vi "Handle Last Ack Core.vi"(4 "error in (no error)":errorcluster, 6 "Last Ack":refnum<class "Last Ack.lvclass">, 7 "Server in":refnum<class "Server.lvclass">) -> (0 "error out":errorcluster, 3 "Server out":refnum<class "Server.lvclass">)   [LabVIEW 2020, in "Server.lvlib" / "Server.lvclass"]
doc: "(<B>Filename</B>: Actor Framework.lvlib:Actor.lvclass:Handle Last Ack Core.vi)\n\nDefines how the caller actor responds to the Last Ack message from a nested actor. The Last Ack message is the final message a nested actor sends to its caller before it shuts down. The message contains information about the final state of the nested actor.\n\nBy default, this method does nothing except return any error the nested actor sent. A descendant class may override this method to define behavior."
uses:
  Server.lvclass
  <vilib>/ActorFramework/LastAck/Last Ack.lvclass
  C:/Program Files/National Instruments/LabVIEW 2020/vi.lib/ActorFramework/Actor/Actor.lvclass
  <vilib>/ActorFramework/Actor/Actor.lvclass/Actor.ctl
  <vilib>/ActorFramework/Message Enqueuer/Message Enqueuer.lvclass/Message Enqueuer.ctl
  Server.lvclass/Server.ctl
  Chat Window Model/Chat Window Model Messages/Update Online List Msg/Update Online List Msg.lvclass/Update Online List Msg.ctl
  Chat Window Model/Chat Window Model Messages/Update Status Log Msg/Update Status Log Msg.lvclass/Update Status Log Msg.ctl
  Server Messages/Enable Controls Msg/Enable Controls Msg.lvclass/Enable Controls Msg.ctl
  <vilib>/ActorFramework/Message Enqueuer/Init from Existing Queue.vi
  <vilib>/ActorFramework/Message Enqueuer/Enqueue.vi
  Chat Window Model/Chat Window Model Messages/Update Online List Msg/Update Online List Msg.lvclass
  C:/Program Files/National Instruments/LabVIEW 2020/vi.lib/ActorFramework/Message/Message.lvclass
  Chat Window Model/Chat Window Model Messages/Update Status Log Msg/Update Status Log Msg.lvclass
  Server Messages/Enable Controls Msg/Enable Controls Msg.lvclass
  <vilib>/ActorFramework/Message Priority Queue/Priority Enqueue.vi
  <vilib>/ActorFramework/Message Enqueuer/Message Enqueuer.lvclass
  <vilib>/ActorFramework/Actor/Actor.lvclass
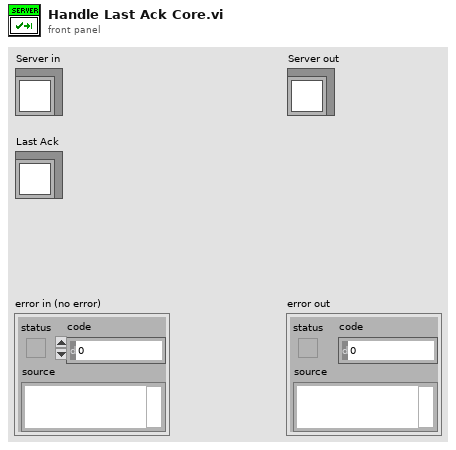
[diagram p1: front panel]
types:
  T1 = enum8{"Enabled", "Disabled", "Disabled and Grayed Out"}
  T2 = map{string, cluster{"Enqueuer":refnum<class "Message Enqueuer.lvclass">, "Status":string}}
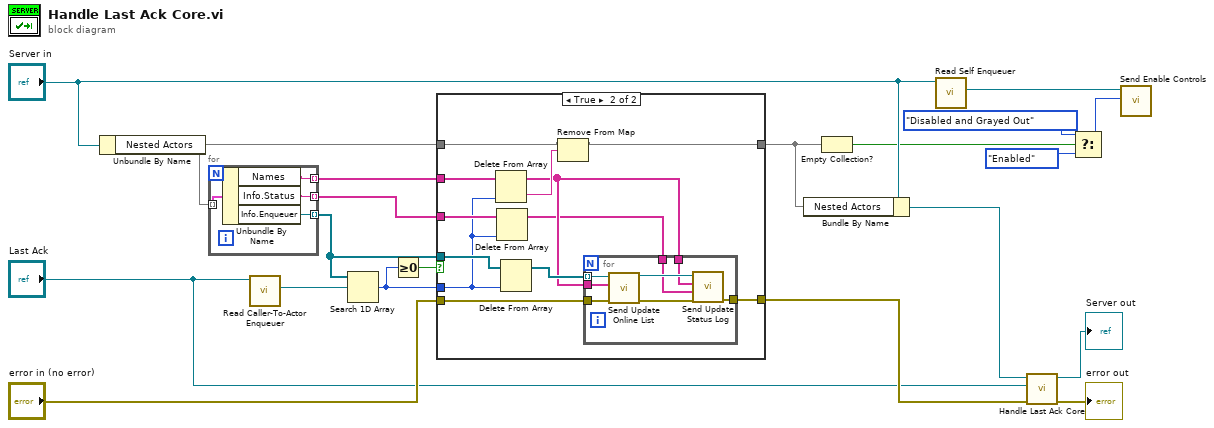
[diagram p0: block diagram]
diagram:
  n1 = Unbundle By Name("Server in") -> ("Nested Actors"=w6:T2)
  n2 = for {
    tunnel: w6 -> [w24] mode=indexing
    tunnel: [w23] -> w5 mode=indexing
    tunnel: [w22] -> w1 mode=indexing
    tunnel: [w21] -> w2 mode=indexing
    n3 = Unbundle By Name(w24) -> ("Names"=w21:string, "Info.Status"=w22:string, "Info.Enqueuer"=w23:refnum<class "Message Enqueuer.lvclass">)
  }
  n4 = call <vilib>:"Read Caller-To-Actor Enqueuer.vi"("Last Ack"="Last Ack") -> ("Caller-to-Actor Enqueuer"=w7:refnum<class "Message Enqueuer.lvclass">)  [unwired: 10 in]
  n5 = Search 1D Array(1D array=w5, element=w7) -> (index of element=w18:i32)  [unwired: 1 in]
  n6 = Greater Or Equal To 0?(x=w18) -> (x >= 0?=w17:bool)
  n7 = case shown="True" w17 {
    tunnel: w5 -> [_ w38]
    tunnel: w18 -> [_ w28]
    tunnel: w2 -> [_ w37]
    tunnel: w6 -> [w26 w33]
    tunnel: [w26 w31] -> w4
    tunnel: "error in (no error)" -> [w25 w35]
    tunnel: [w25 w34] -> w14
    tunnel: w1 -> [_ w29]
    frame False {
    }
    frame True {
      n8 = Delete From Array(array=w37, index=w28) -> (deleted portion=w32:string, array with subset deleted=w30:string[])  [unwired: 1 in]
      n9 = Delete From Array(array=w29, index=w28) -> (array with subset deleted=w27:string[])  [unwired: 1 in, 1 out]
      n10 = Delete From Array(array=w38, index=w28) -> (array with subset deleted=w36:refnum<class "Message Enqueuer.lvclass">[])  [unwired: 1 in, 1 out]
      n11 = Remove From Map(10:w32, 11:w33) -> (3:w31:T2)  [unwired: 2 out]
      n12 = for {
        tunnel: w36 -> [w45] mode=indexing
        tunnel: w30 -> [w46]
        tunnel: w27 -> [w42]
        tunnel: w30 -> [w41]
        tunnel: w35 -> [w40]
        tunnel: [w39] -> w34
        n13 = call "Send Update Online List.vi"("error in (no error)"=w40, "Online Users"=w46, "Message Enqueuer in"=w45) -> ("error out"=w43:errorcluster, "Message Enqueuer out"=w44:refnum<class "Message Enqueuer.lvclass">)  [unwired: 7 in]
        n14 = call "Send Update Status Log.vi"("error in (no error)"=w43, "Status List"=w42, "Names"=w41, "Message Enqueuer in"=w44) -> ("error out"=w39:errorcluster)  [unwired: 6 in, 1 out]
      }
    }
  }
  n15 = Bundle By Name(cluster="Server in", "Nested Actors"=w4) -> (w16:refnum<class "Server.lvclass">)
  n16 = Empty Collection?(1:w4) -> (0:w3:bool)
  n17 = call <vilib>:"Read Self Enqueuer.vi"("Actor"="Server in") -> ("Self Enqueuer"=w12:refnum<class "Message Enqueuer.lvclass">)  [unwired: 10 in]
  n18 = call-parent "Handle Last Ack Core.vi"("error in (no error)"=w14, "Last Ack"="Last Ack", "Actor in"=w16) -> ("error out"=→"error out":errorcluster, "Actor out"=→"Server out":refnum<class "Server.lvclass">)  [unwired: 3 in]
  n19 = Select(t=T1."Disabled and Grayed Out" ("Disabled"), s=w3, f=T1."Enabled" ("Disabled")) -> (s? t:f=w11:T1)
  n20 = call "Send Enable Controls.vi"("Disabled"=w11, "Message Enqueuer in"=w12) -> ()  [unwired: 8 in, 2 out]
